vi "Generate Letter Coordenates.vi"(8 "Error In":errorcluster, 11 "Letter":string) -> (0 "Error Out":errorcluster, 2 "Width":i32, 3 "Element To Display":T1[](array[typedef]))   [LabVIEW 2019, in "String.lvclass"]
uses:
  String.lvclass
  Display Utilities/Public/Controls/2D Coordenates.ctl
  Display Utilities/Display Utilities.lvlib
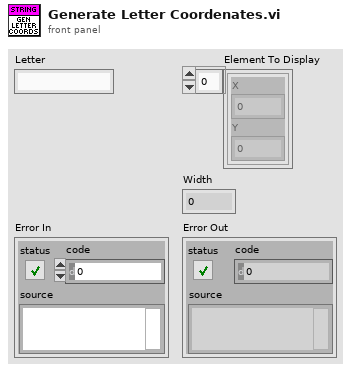
[diagram p1: front panel]
types:
  T1 = typedef "Display Utilities.lvlib/2D Coordenates.ctl" = cluster{"X":i32, "Y":i32}
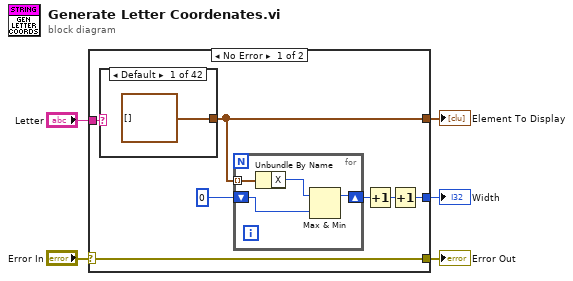
[diagram p0: block diagram]
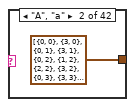
[diagram p2: hidden frame]
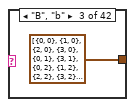
[diagram p3: hidden frame]
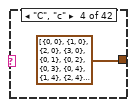
[diagram p4: hidden frame]
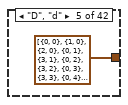
[diagram p5: hidden frame]
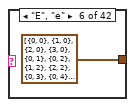
[diagram p6: hidden frame]
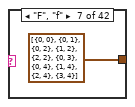
[diagram p7: hidden frame]
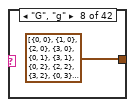
[diagram p8: hidden frame]
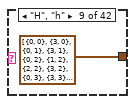
[diagram p9: hidden frame]
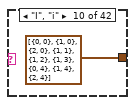
[diagram p10: hidden frame]
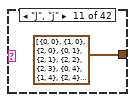
[diagram p11: hidden frame]
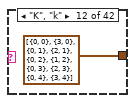
[diagram p12: hidden frame]
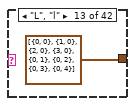
[diagram p13: hidden frame]
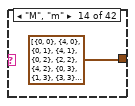
[diagram p14: hidden frame]
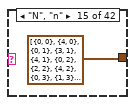
[diagram p15: hidden frame]
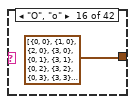
[diagram p16: hidden frame]
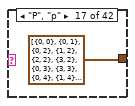
[diagram p17: hidden frame]
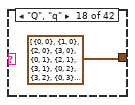
[diagram p18: hidden frame]
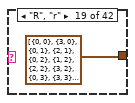
[diagram p19: hidden frame]
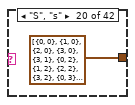
[diagram p20: hidden frame]
diagram:
  n1 = case shown="No Error" "Error In" {
    selector: "Error In" -> [w11 w61]
    tunnel: [w11 w61] -> w4
    tunnel: "Letter" -> [w12 _]
    tunnel: [w6 T1[] [] ("Coordenates")] -> w2
    tunnel: [w7 0 ("X")] -> w1
    frame No Error {
      n2 = case shown="Default" w12 {
        tunnel: [T1[] [] ("Element To Display") T1[] [{"X"=0, "Y"=0}, {"X"=3, "Y"=0}, {"X"=0, "Y"=1}, {"X"=3, "Y"=1}, {"X"=0, "Y"=2}, {"X"=1, "Y"=2}, {"X"=2, "Y"=2}, {"X"=3, "Y"=2}, {"X"=0, "Y"=3}, {"X"=3, "Y"=3}, {"X"=0, "Y"=4}, {"X"=1, "Y"=4}, {"X"=2, "Y"=4}, {"X"=3, "Y"=4}] ("Coordenates") T1[] [{"X"=0, "Y"=0}, {"X"=1, "Y"=0}, {"X"=2, "Y"=0}, {"X"=3, "Y"=0}, {"X"=0, "Y"=1}, {"X"=3, "Y"=1}, {"X"=0, "Y"=2}, {"X"=1, "Y"=2}, {"X"=2, "Y"=2}, {"X"=3, "Y"=2}, {"X"=0, "Y"=3}, {"X"=2, "Y"=3}, {"X"=0, "Y"=4}, {"X"=1, "Y"=4}, {"X"=2, "Y"=4}] ("Coordenates") T1[] [{"X"=0, "Y"=0}, {"X"=1, "Y"=0}, {"X"=2, "Y"=0}, {"X"=3, "Y"=0}, {"X"=0, "Y"=1}, {"X"=0, "Y"=2}, {"X"=0, "Y"=3}, {"X"=0, "Y"=4}, {"X"=1, "Y"=4}, {"X"=2, "Y"=4}, {"X"=3, "Y"=4}] ("Coordenates") T1[] [{"X"=0, "Y"=0}, {"X"=1, "Y"=0}, {"X"=2, "Y"=0}, {"X"=0, "Y"=1}, {"X"=3, "Y"=1}, {"X"=0, "Y"=2}, {"X"=3, "Y"=2}, {"X"=0, "Y"=3}, {"X"=3, "Y"=3}, {"X"=0, "Y"=4}, {"X"=1, "Y"=4}, {"X"=2, "Y"=4}] ("Coordenates") T1[] [{"X"=0, "Y"=0}, {"X"=1, "Y"=0}, {"X"=2, "Y"=0}, {"X"=3, "Y"=0}, {"X"=0, "Y"=1}, {"X"=0, "Y"=2}, {"X"=1, "Y"=2}, {"X"=2, "Y"=2}, {"X"=0, "Y"=3}, {"X"=0, "Y"=4}, {"X"=1, "Y"=4}, {"X"=2, "Y"=4}, {"X"=3, "Y"=4}] ("Coordenates") T1[] [{"X"=0, "Y"=0}, {"X"=0, "Y"=1}, {"X"=0, "Y"=2}, {"X"=1, "Y"=2}, {"X"=2, "Y"=2}, {"X"=0, "Y"=3}, {"X"=0, "Y"=4}, {"X"=1, "Y"=4}, {"X"=2, "Y"=4}, {"X"=3, "Y"=4}] ("Coordenates") T1[] [{"X"=0, "Y"=0}, {"X"=1, "Y"=0}, {"X"=2, "Y"=0}, {"X"=3, "Y"=0}, {"X"=0, "Y"=1}, {"X"=3, "Y"=1}, {"X"=0, "Y"=2}, {"X"=2, "Y"=2}, {"X"=3, "Y"=2}, {"X"=0, "Y"=3}, {"X"=0, "Y"=4}, {"X"=1, "Y"=4}, {"X"=2, "Y"=4}, {"X"=3, "Y"=4}] ("Coordenates") T1[] [{"X"=0, "Y"=0}, {"X"=3, "Y"=0}, {"X"=0, "Y"=1}, {"X"=3, "Y"=1}, {"X"=0, "Y"=2}, {"X"=1, "Y"=2}, {"X"=2, "Y"=2}, {"X"=3, "Y"=2}, {"X"=0, "Y"=3}, {"X"=3, "Y"=3}, {"X"=0, "Y"=4}, {"X"=3, "Y"=4}] ("Coordenates") T1[] [{"X"=0, "Y"=0}, {"X"=1, "Y"=0}, {"X"=2, "Y"=0}, {"X"=1, "Y"=1}, {"X"=1, "Y"=2}, {"X"=1, "Y"=3}, {"X"=0, "Y"=4}, {"X"=1, "Y"=4}, {"X"=2, "Y"=4}] ("Coordenates") T1[] [{"X"=0, "Y"=0}, {"X"=1, "Y"=0}, {"X"=2, "Y"=0}, {"X"=0, "Y"=1}, {"X"=2, "Y"=1}, {"X"=2, "Y"=2}, {"X"=2, "Y"=3}, {"X"=0, "Y"=4}, {"X"=1, "Y"=4}, {"X"=2, "Y"=4}, {"X"=3, "Y"=4}] ("Coordenates") T1[] [{"X"=0, "Y"=0}, {"X"=3, "Y"=0}, {"X"=0, "Y"=1}, {"X"=2, "Y"=1}, {"X"=0, "Y"=2}, {"X"=1, "Y"=2}, {"X"=0, "Y"=3}, {"X"=2, "Y"=3}, {"X"=0, "Y"=4}, {"X"=3, "Y"=4}] ("Coordenates") T1[] [{"X"=0, "Y"=0}, {"X"=1, "Y"=0}, {"X"=2, "Y"=0}, {"X"=3, "Y"=0}, {"X"=0, "Y"=1}, {"X"=0, "Y"=2}, {"X"=0, "Y"=3}, {"X"=0, "Y"=4}] ("Coordenates") T1[] [{"X"=0, "Y"=0}, {"X"=4, "Y"=0}, {"X"=0, "Y"=1}, {"X"=4, "Y"=1}, {"X"=0, "Y"=2}, {"X"=2, "Y"=2}, {"X"=4, "Y"=2}, {"X"=0, "Y"=3}, {"X"=1, "Y"=3}, {"X"=3, "Y"=3}, {"X"=4, "Y"=3}, {"X"=0, "Y"=4}, {"X"=4, "Y"=4}] ("Coordenates") T1[] [{"X"=0, "Y"=0}, {"X"=4, "Y"=0}, {"X"=0, "Y"=1}, {"X"=3, "Y"=1}, {"X"=4, "Y"=1}, {"X"=0, "Y"=2}, {"X"=2, "Y"=2}, {"X"=4, "Y"=2}, {"X"=0, "Y"=3}, {"X"=1, "Y"=3}, {"X"=4, "Y"=3}, {"X"=0, "Y"=4}, {"X"=4, "Y"=4}] ("Coordenates") T1[] [{"X"=0, "Y"=0}, {"X"=1, "Y"=0}, {"X"=2, "Y"=0}, {"X"=3, "Y"=0}, {"X"=0, "Y"=1}, {"X"=3, "Y"=1}, {"X"=0, "Y"=2}, {"X"=3, "Y"=2}, {"X"=0, "Y"=3}, {"X"=3, "Y"=3}, {"X"=0, "Y"=4}, {"X"=1, "Y"=4}, {"X"=2, "Y"=4}, {"X"=3, "Y"=4}] ("Coordenates") T1[] [{"X"=0, "Y"=0}, {"X"=0, "Y"=1}, {"X"=0, "Y"=2}, {"X"=1, "Y"=2}, {"X"=2, "Y"=2}, {"X"=3, "Y"=2}, {"X"=0, "Y"=3}, {"X"=3, "Y"=3}, {"X"=0, "Y"=4}, {"X"=1, "Y"=4}, {"X"=2, "Y"=4}, {"X"=3, "Y"=4}] ("Coordenates") T1[] [{"X"=0, "Y"=0}, {"X"=1, "Y"=0}, {"X"=2, "Y"=0}, {"X"=3, "Y"=0}, {"X"=0, "Y"=1}, {"X"=2, "Y"=1}, {"X"=3, "Y"=1}, {"X"=0, "Y"=2}, {"X"=3, "Y"=2}, {"X"=0, "Y"=3}, {"X"=3, "Y"=3}, {"X"=0, "Y"=4}, {"X"=1, "Y"=4}, {"X"=2, "Y"=4}, {"X"=3, "Y"=4}] ("Coordenates") T1[] [{"X"=0, "Y"=0}, {"X"=3, "Y"=0}, {"X"=0, "Y"=1}, {"X"=2, "Y"=1}, {"X"=0, "Y"=2}, {"X"=1, "Y"=2}, {"X"=2, "Y"=2}, {"X"=3, "Y"=2}, {"X"=0, "Y"=3}, {"X"=3, "Y"=3}, {"X"=0, "Y"=4}, {"X"=1, "Y"=4}, {"X"=2, "Y"=4}, {"X"=3, "Y"=4}] ("Coordenates") T1[] [{"X"=0, "Y"=0}, {"X"=1, "Y"=0}, {"X"=2, "Y"=0}, {"X"=3, "Y"=0}, {"X"=3, "Y"=1}, {"X"=0, "Y"=2}, {"X"=1, "Y"=2}, {"X"=2, "Y"=2}, {"X"=3, "Y"=2}, {"X"=0, "Y"=3}, {"X"=0, "Y"=4}, {"X"=1, "Y"=4}, {"X"=2, "Y"=4}, {"X"=3, "Y"=4}] ("Coordenates") T1[] [{"X"=1, "Y"=0}, {"X"=1, "Y"=1}, {"X"=1, "Y"=2}, {"X"=1, "Y"=3}, {"X"=0, "Y"=4}, {"X"=1, "Y"=4}, {"X"=2, "Y"=4}] ("Coordenates") T1[] [{"X"=0, "Y"=0}, {"X"=1, "Y"=0}, {"X"=2, "Y"=0}, {"X"=3, "Y"=0}, {"X"=0, "Y"=1}, {"X"=3, "Y"=1}, {"X"=0, "Y"=2}, {"X"=3, "Y"=2}, {"X"=0, "Y"=3}, {"X"=3, "Y"=3}, {"X"=0, "Y"=4}, {"X"=3, "Y"=4}] ("Coordenates") T1[] [{"X"=1, "Y"=0}, {"X"=2, "Y"=0}, {"X"=1, "Y"=1}, {"X"=2, "Y"=1}, {"X"=0, "Y"=2}, {"X"=3, "Y"=2}, {"X"=0, "Y"=3}, {"X"=3, "Y"=3}, {"X"=0, "Y"=4}, {"X"=3, "Y"=4}] ("Coordenates") T1[] [{"X"=0, "Y"=0}, {"X"=4, "Y"=0}, {"X"=0, "Y"=1}, {"X"=1, "Y"=1}, {"X"=3, "Y"=1}, {"X"=4, "Y"=1}, {"X"=0, "Y"=2}, {"X"=2, "Y"=2}, {"X"=4, "Y"=2}, {"X"=0, "Y"=3}, {"X"=4, "Y"=3}, {"X"=0, "Y"=4}, {"X"=4, "Y"=4}] ("Coordenates") T1[] [{"X"=0, "Y"=0}, {"X"=2, "Y"=0}, {"X"=0, "Y"=1}, {"X"=2, "Y"=1}, {"X"=1, "Y"=2}, {"X"=0, "Y"=3}, {"X"=2, "Y"=3}, {"X"=0, "Y"=4}, {"X"=2, "Y"=4}] ("Coordenates") T1[] [{"X"=1, "Y"=0}, {"X"=1, "Y"=1}, {"X"=1, "Y"=2}, {"X"=0, "Y"=3}, {"X"=2, "Y"=3}, {"X"=0, "Y"=4}, {"X"=2, "Y"=4}] ("Coordenates") T1[] [{"X"=0, "Y"=0}, {"X"=1, "Y"=0}, {"X"=2, "Y"=0}, {"X"=0, "Y"=1}, {"X"=1, "Y"=2}, {"X"=2, "Y"=3}, {"X"=0, "Y"=4}, {"X"=1, "Y"=4}, {"X"=2, "Y"=4}] ("Coordenates") T1[] [{"X"=0, "Y"=0}, {"X"=1, "Y"=0}, {"X"=2, "Y"=0}, {"X"=0, "Y"=1}, {"X"=2, "Y"=1}, {"X"=0, "Y"=2}, {"X"=2, "Y"=2}, {"X"=0, "Y"=3}, {"X"=2, "Y"=3}, {"X"=0, "Y"=4}, {"X"=1, "Y"=4}, {"X"=2, "Y"=4}] ("Coordenates") T1[] [{"X"=1, "Y"=0}, {"X"=1, "Y"=1}, {"X"=1, "Y"=2}, {"X"=1, "Y"=3}, {"X"=0, "Y"=4}, {"X"=1, "Y"=4}] ("Coordenates") T1[] [{"X"=0, "Y"=0}, {"X"=1, "Y"=0}, {"X"=2, "Y"=0}, {"X"=0, "Y"=1}, {"X"=0, "Y"=2}, {"X"=1, "Y"=2}, {"X"=2, "Y"=2}, {"X"=2, "Y"=3}, {"X"=0, "Y"=4}, {"X"=1, "Y"=4}, {"X"=2, "Y"=4}] ("Coordenates") T1[] [{"X"=0, "Y"=0}, {"X"=1, "Y"=0}, {"X"=2, "Y"=0}, {"X"=2, "Y"=1}, {"X"=0, "Y"=2}, {"X"=1, "Y"=2}, {"X"=2, "Y"=2}, {"X"=2, "Y"=3}, {"X"=0, "Y"=4}, {"X"=1, "Y"=4}, {"X"=2, "Y"=4}] ("Coordenates") T1[] [{"X"=2, "Y"=0}, {"X"=2, "Y"=1}, {"X"=0, "Y"=2}, {"X"=1, "Y"=2}, {"X"=2, "Y"=2}, {"X"=0, "Y"=3}, {"X"=2, "Y"=3}, {"X"=0, "Y"=4}, {"X"=2, "Y"=4}] ("Coordenates") T1[] [{"X"=0, "Y"=0}, {"X"=1, "Y"=0}, {"X"=2, "Y"=0}, {"X"=2, "Y"=1}, {"X"=0, "Y"=2}, {"X"=1, "Y"=2}, {"X"=2, "Y"=2}, {"X"=0, "Y"=3}, {"X"=0, "Y"=4}, {"X"=1, "Y"=4}, {"X"=2, "Y"=4}] ("Coordenates") T1[] [{"X"=0, "Y"=0}, {"X"=1, "Y"=0}, {"X"=2, "Y"=0}, {"X"=0, "Y"=1}, {"X"=2, "Y"=1}, {"X"=0, "Y"=2}, {"X"=1, "Y"=2}, {"X"=2, "Y"=2}, {"X"=0, "Y"=3}, {"X"=0, "Y"=4}, {"X"=1, "Y"=4}, {"X"=2, "Y"=4}] ("Coordenates") T1[] [{"X"=2, "Y"=0}, {"X"=2, "Y"=1}, {"X"=2, "Y"=2}, {"X"=2, "Y"=3}, {"X"=0, "Y"=4}, {"X"=1, "Y"=4}, {"X"=2, "Y"=4}] ("Coordenates") T1[] [{"X"=0, "Y"=0}, {"X"=1, "Y"=0}, {"X"=2, "Y"=0}, {"X"=0, "Y"=1}, {"X"=2, "Y"=1}, {"X"=0, "Y"=2}, {"X"=1, "Y"=2}, {"X"=2, "Y"=2}, {"X"=0, "Y"=3}, {"X"=2, "Y"=3}, {"X"=0, "Y"=4}, {"X"=1, "Y"=4}, {"X"=2, "Y"=4}] ("Coordenates") T1[] [{"X"=2, "Y"=0}, {"X"=2, "Y"=1}, {"X"=0, "Y"=2}, {"X"=1, "Y"=2}, {"X"=2, "Y"=2}, {"X"=0, "Y"=3}, {"X"=2, "Y"=3}, {"X"=0, "Y"=4}, {"X"=1, "Y"=4}, {"X"=2, "Y"=4}] ("Coordenates") T1[] [{"X"=0, "Y"=1}, {"X"=0, "Y"=3}] ("Coordenates") T1[] [{"X"=0, "Y"=0}] ("Coordenates") T1[] [{"X"=1, "Y"=0}, {"X"=1, "Y"=1}, {"X"=2, "Y"=2}, {"X"=0, "Y"=3}, {"X"=2, "Y"=3}, {"X"=0, "Y"=4}, {"X"=1, "Y"=4}, {"X"=2, "Y"=4}] ("Coordenates") T1[] [{"X"=0, "Y"=0}, {"X"=0, "Y"=2}, {"X"=0, "Y"=3}, {"X"=0, "Y"=4}] ("Coordenates") T1[] [{"X"=0, "Y"=2}, {"X"=1, "Y"=2}] ("Coordenates")] -> w6
        frame Default {
        }
        frame "A", "a" {
        }
        frame "B", "b" {
        }
        frame "C", "c" {
        }
        frame "D", "d" {
        }
        frame "E", "e" {
        }
        frame "F", "f" {
        }
        frame "G", "g" {
        }
        frame "H", "h" {
        }
        frame "I", "i" {
        }
        frame "J", "j" {
        }
        frame "K", "k" {
        }
        frame "L", "l" {
        }
        frame "M", "m" {
        }
        frame "N", "n" {
        }
        frame "O", "o" {
        }
        frame "P", "p" {
        }
        frame "Q", "q" {
        }
        frame "R", "r" {
        }
        frame "S", "s" {
        }
        frame "T", "t" {
        }
        frame "U", "u" {
        }
        frame "V", "v" {
        }
        frame "W", "w" {
        }
        frame "X", "x" {
        }
        frame "Y", "y" {
        }
        frame "Z", "z" {
        }
        frame "0" {
        }
        frame "1" {
        }
        frame "2" {
        }
        frame "3" {
        }
        frame "4" {
        }
        frame "5" {
        }
        frame "6" {
        }
        frame "7" {
        }
        frame "8" {
        }
        frame "9" {
        }
        frame ":" {
        }
        frame "." {
        }
        frame "?" {
        }
        frame "!" {
        }
        frame "-" {
        }
      }
      n3 = for {
        tunnel: w6 -> [w56] mode=indexing
        shift-right: [w57] -> w9
        shift-left: 0 ("X") -> [w58]
        n4 = Unbundle By Name(w56) -> ("X"=w55:i32)
        n5 = Max & Min(x=w55, y=w58) -> (max(x,y)=w57:i32)  [unwired: 1 out]
      }
      n6 = Increment(x=w9) -> (x+1=w8:i32)
      n7 = Increment(x=w8) -> (x+1=w7:i32)
    }
    frame Error {
    }
  }
  "Error Out" <- w4
  "Element To Display" <- w2
  "Width" <- w1
